vi "Get State Queue Ref.vi"(8 "error in (no error)":errorcluster) -> (0 "error out":errorcluster, 3 "queue out":refnum<queue>)   [LabVIEW 2014]
uses:
  Controls/State Typedef.ctl
  Controls/StateControl.ctl
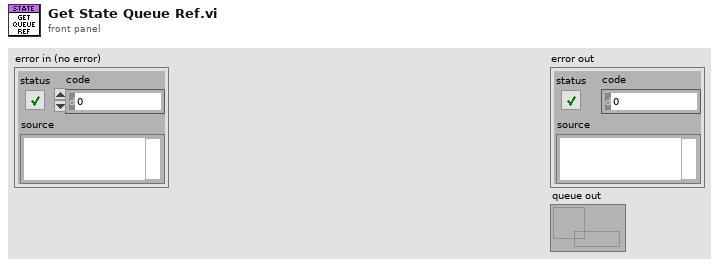
[diagram p1: front panel]
types:
  T1 = typedef "State Typedef.ctl" = cluster{"State":T2, "Data":variant}
  T2 = typedef "StateControl.ctl" = enum16{"WAIT FOR EVENT", "GET HEALTH", "SCAN", "RESET", "EXIT"}
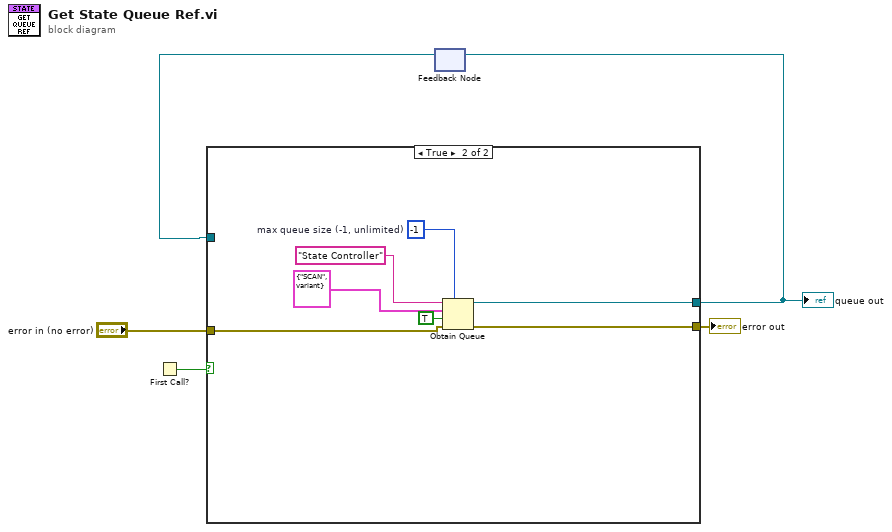
[diagram p0: block diagram]
diagram:
  n1 = First Call?() -> (First Call?: T/F=w5:bool)
  n2 = feedback #1() -> (w1:refnum<queue>)  [unwired: 1 in]
  n3 = case shown="True" w5 {
    tunnel: "error in (no error)" -> [w6 w10]
    tunnel: [w6 w9] -> w3
    tunnel: [w7 w8] -> w2
    tunnel: w1 -> [w7 _]
    frame False {
    }
    frame True {
      w13 = -1  # max queue size (-1, unlimited)
      n4 = Obtain Queue(max queue size (-1, unlimited)=w13, name (unnamed)="State Controller", element data type=T1 {"State"=enum."SCAN", "Data"=variant} ("State Control"), create if not found? (T)=TRUE, error in (no error)=w10) -> (queue out=w8:refnum<queue>, error out=w9:errorcluster)  [unwired: 1 out]
    }
  }
  "error out" <- w3
  "queue out" <- w2
  n5 = feedback-in #1(w2) -> ()
